vi "_RT Get Lens Configuration.vi"(5 "Name":string, 7 "Channel #":u8) -> (0 "Found":bool, 1 "Config Row#":i32, 3 "Lens Configuration":T1)   [LabVIEW 2015]
uses:
  Type/_RT Configuration 2.ctl
  _RT Global.vi
panel:
  # "Get lens properties from a configuration table by ch# or name"
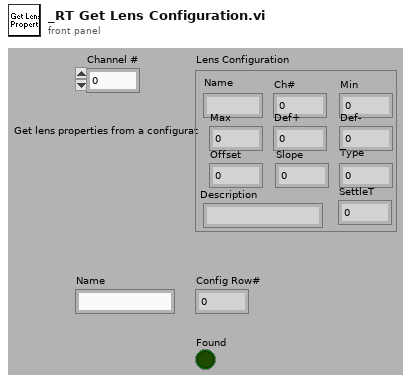
[diagram p1: front panel]
types:
  T1 = typedef "_RT Configuration 2.ctl" = cluster{"Name":string, "Ch#":u8, "Min":dbl, "Max":dbl, "Def+":dbl, "Def-":dbl, "Offset":dbl, "Slope":dbl, "Type":u8, "Description":string, "SettleT":dbl}
  T2 = typedef "_RT Instrument 2.ctl" = cluster{"Table":T1[], "Instrument":string[]}
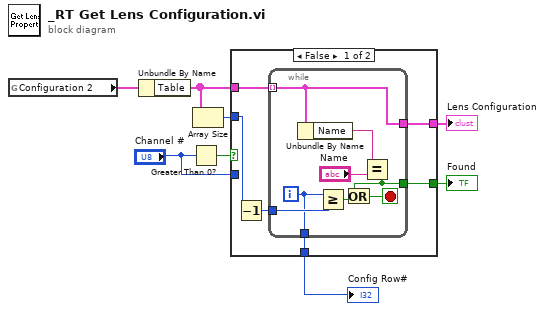
[diagram p0: block diagram]
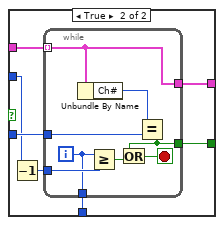
[diagram p2: hidden frame]
diagram:
  n1 = global read "_RT Global.vi" "Configuration 2"() -> (w6:T2)
  n2 = Unbundle By Name(w6) -> ("Table"=w5:T1[])
  n3 = Greater Than 0?(x="Channel #") -> (x > 0?=w8:bool)
  n4 = Array Size(array=w5) -> (size(s)=w4:i32)
  n5 = case shown="False" w8 {
    tunnel: w5 -> [w13 w29]
    tunnel: [w14 w28] -> w3
    tunnel: "Channel #" -> [_ w27]
    tunnel: w4 -> [w12 w26]
    tunnel: [w10 w24] -> w2
    tunnel: [w9 w23] -> w1
    frame False {
      n6 = Decrement(x=w12) -> (x-1=w11:i32)
      n7 = while {
        tunnel: w13 -> [w19] mode=indexing
        tunnel: [w19] -> w14
        tunnel: w11 -> [w20]
        tunnel: [w16] -> w10
        tunnel: [w15] -> w9
        i -> [w16]
        stop <- w22 stop-if-true
        n8 = Unbundle By Name(w19) -> ("Name"=w18:string)
        n9 = Greater Or Equal?(x=w16, y=w20) -> (x >= y?=w21:bool)
        n10 = Equal?(x=w18, y="Name") -> (x = y?=w15:bool)
        n11 = Or(x=w15, y=w21) -> (x .or. y?=w22:bool)
      }
    }
    frame True {
      n12 = Decrement(x=w26) -> (x-1=w25:i32)
      n13 = while {
        tunnel: w29 -> [w33] mode=indexing
        tunnel: [w33] -> w28
        tunnel: w27 -> [w37]
        tunnel: w25 -> [w34]
        tunnel: [w31] -> w24
        tunnel: [w30] -> w23
        i -> [w31]
        stop <- w36 stop-if-true
        n14 = Unbundle By Name(w33) -> ("Ch#"=w32:u8)
        n15 = Greater Or Equal?(x=w31, y=w34) -> (x >= y?=w35:bool)
        n16 = Equal?(x=w32, y=w37) -> (x = y?=w30:bool)
        n17 = Or(x=w30, y=w35) -> (x .or. y?=w36:bool)
      }
    }
  }
  "Lens Configuration" <- w3
  "Config Row#" <- w2
  "Found" <- w1
